vi "IsInput.vi"(6 "error in":errorcluster, 9 "ControlTerminal in":refnum<class "ControlTerminal.lvclass">) -> (0 "error out":errorcluster, 2 "input":bool, 3 "ControlTerminal out":refnum<class "ControlTerminal.lvclass">)   [LabVIEW 2014, in "Raspberry Pi Compatible Compiler for LabVIEW.lvlib" / "ControlTerminal.lvclass"]
uses:
  ControlTerminal.lvclass
  Terminal/Terminal.lvclass
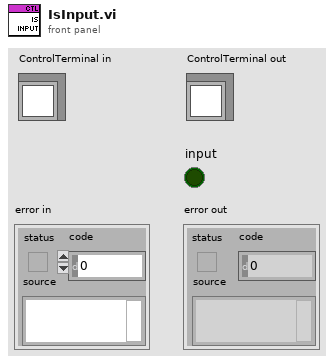
[diagram p1: front panel]
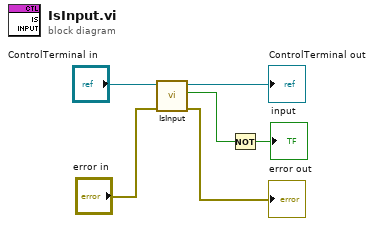
[diagram p0: block diagram]
diagram:
  n1 = call-parent "IsInput.vi"("error in"="error in", "Terminal in"="ControlTerminal in") -> ("error out"=→"error out":errorcluster, "input"=w5:bool, "Terminal out"=→"ControlTerminal out":refnum<class "ControlTerminal.lvclass">)  [unwired: 5 in]
  n2 = Not(x=w5) -> (.not. x?=→"input":bool)
